vi "GET_Click_Coords.vi"(0 "Screen coords in, pix":T2, 1 "Size of the image":T1={"Numeric Control"=480.0, "Numeric Control"=480.0}, 5 "Pixels per mm":dbl=2.0) -> (4 "Click coords, mm":T1)   [LabVIEW 2018, in "Tracker.lvlib"]
uses:
  Tracker.lvlib
  <vilib>/Utility/miscctls.llb/LVPoint32TypeDef.ctl
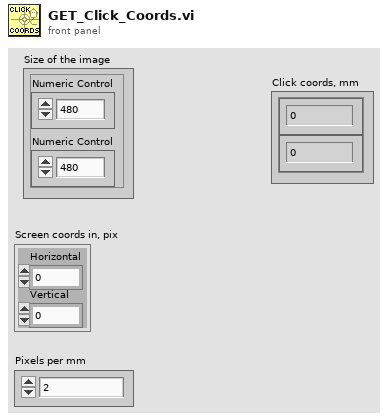
[diagram p1: front panel]
types:
  T1 = cluster{"Numeric Control":dbl, "Numeric Control":dbl}
  T2 = typedef "LVPoint32TypeDef.ctl" = cluster{"Horizontal":i32, "Vertical":i32}
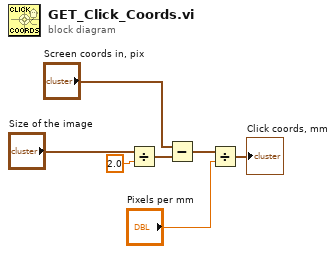
[diagram p0: block diagram]
diagram:
  n1 = Divide(x="Size of the image", y=2.0) -> (x/y=w1:T1)
  n2 = Subtract(x="Screen coords in, pix", y=w1) -> (x-y=w6:cluster{dbl, dbl})
  n3 = Divide(x=w6, y="Pixels per mm") -> (x/y=→"Click coords, mm":cluster{dbl, dbl})
